vi "limit.vi"(1 "Limit":dbl, 2 "Input":dbl) -> (0 "Output":dbl)   [LabVIEW 2014]
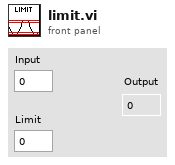
[diagram p1: front panel]
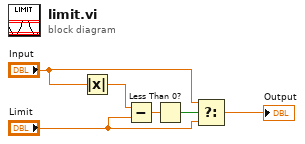
[diagram p0: block diagram]
diagram:
  n1 = Absolute Value(x="Input") -> (abs(x)=w6:dbl)
  n2 = Subtract(x=w6, y="Limit") -> (x-y=w5:dbl)
  n3 = Less Than 0?(x=w5) -> (x < 0?=w4:bool)
  n4 = Select(t="Input", s=w4, f="Limit") -> (s? t:f=→"Output":dbl)
